vi "Destroy.vi"(0 "Universal Robot in":refnum<class "Universal Robot.lvclass">, 5 "error in (no error)":errorcluster) -> (14 "Universal Robot out":refnum<class "Universal Robot.lvclass">, 19 "error out":errorcluster)   [LabVIEW 2019, in "Universal Robot.lvclass"]
uses:
  Universal Robot.lvclass
  Universal Robot.lvclass/Universal Robot.ctl
  Client Interfaces/Dashboard Server/Dashboard Server.lvclass
  Client Interfaces/Socket Communication/Socket Communication.lvclass
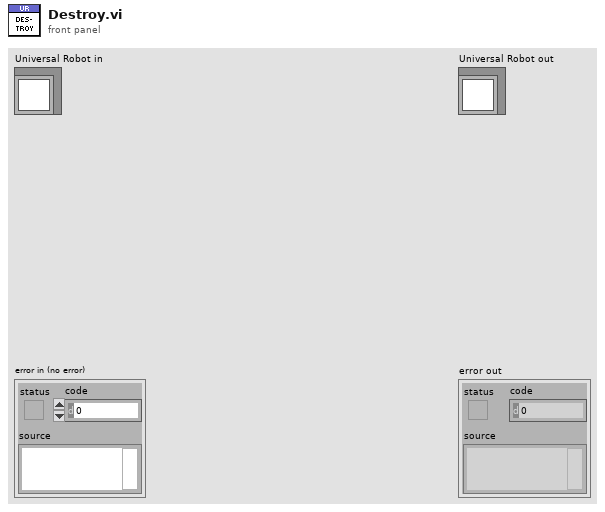
[diagram p1: front panel]
types:
  T1 = typedef "Semaphore RefNum" = refnum<k1>
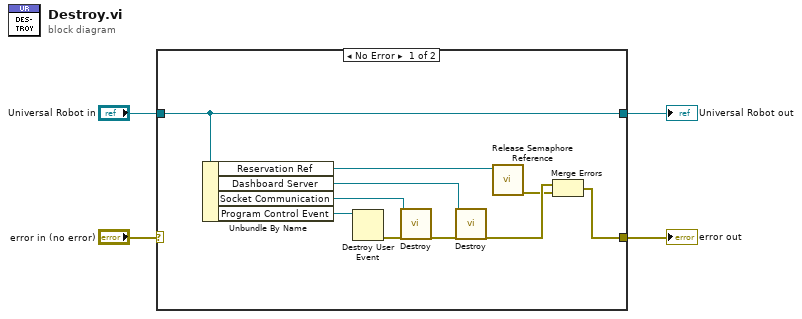
[diagram p0: block diagram]
diagram:
  n1 = case shown="No Error" "error in (no error)" {
    selector: "error in (no error)" -> [_ w16]
    tunnel: [w5 w16] -> w3
    tunnel: [w14 w15] -> w1
    tunnel: "Universal Robot in" -> [w14 w15]
    frame No Error {
      n2 = Unbundle By Name(w14) -> ("Reservation Ref"=w8:T1, "Dashboard Server"=w9:refnum<class "Dashboard Server.lvclass">, "Socket Communication"=w11:refnum<class "Socket Communication.lvclass">, "Program Control Event"=w13:refnum<user-event>)
      n3 = Destroy User Event(user event=w13) -> (error out=w12:errorcluster)  [unwired: 1 in]
      n4 = call-dynamic "Destroy.vi"("Socket Communication in"=w11, "error in (no error)"=w12) -> ("error out"=w10:errorcluster)  [unwired: 16 in, 1 out]
      n5 = call-dynamic "Destroy.vi"("Dashboard Server in"=w9, "error in (no error)"=w10) -> ("error out"=w7:errorcluster)  [unwired: 16 in, 1 out]
      n6 = call <vilib>:"Release Semaphore Reference.vi"("semaphore"=w8) -> ("error out"=w6:errorcluster)  [unwired: 9 in, 1 out]
      n7 = Merge Errors(w7, w6) -> (w5:errorcluster)
    }
    frame Error {
    }
  }
  "error out" <- w3
  "Universal Robot out" <- w1
